vi "sub_calibrate sensor data.vi"(1 "Sensor Column":i32, 2 "Raw Data":dbl) -> (0 "Calibrated Data":dbl)   [LabVIEW 2021]
uses:
  globalvariables.vi
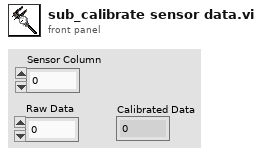
[diagram p1: front panel]
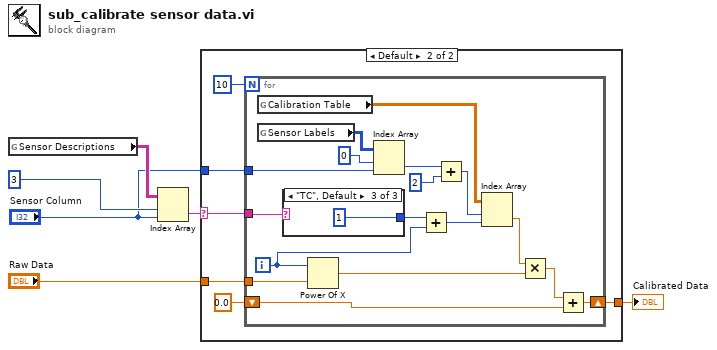
[diagram p0: block diagram]
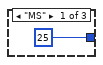
[diagram p3: hidden frame]
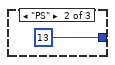
[diagram p4: hidden frame]
diagram:
  n1 = global read "globalvariables.vi" "Sensor Descriptions"() -> (w3:string[][])
  n2 = Index Array(array=w3, index (row)=3, index (col)="Sensor Column") -> (element=w1:string)
  n3 = case shown="Default" w1 {
    selector: w1 -> [_ w9]
    tunnel: [w7 w12] -> w6
    tunnel: "Raw Data" -> [w7 w10]
    tunnel: "Sensor Column" -> [_ w11]
    frame "TM" {
    }
    frame Default {
      n4 = for {
        N: 10 -> [_]
        shift-right: [w30] -> w12
        shift-left: 0.0 -> [w29]
        tunnel: w10 -> [w28]
        tunnel: w11 -> [w27]
        tunnel: w9 -> [w16]
        i -> [w14]
        n5 = global read "globalvariables.vi" "Calibration Table"() -> (w22:dbl[][])
        n6 = global read "globalvariables.vi" "Sensor Labels"() -> (w23:i32[][])
        n7 = case shown="\"TC\", Default" w16 {
          tunnel: [25 13 1] -> w15
          frame "MS" {
          }
          frame "PS" {
          }
          frame "TC", Default {
          }
        }
        n8 = Power Of X(1:w28, 2:w14) -> (0:w26:dbl)
        n9 = Index Array(array=w23, index (row)=0, index (col)=w27) -> (element=w18:i32)
        n10 = Add(x=w15, y=w14) -> (x+y=w20:i32)
        n11 = Add(x=w18, y=2) -> (x+y=w19:i32)
        n12 = Index Array(array=w22, index (row)=w19, index (col)=w20) -> (element=w24:dbl)
        n13 = Multiply(x=w24, y=w26) -> (x*y=w25:dbl)
        n14 = Add(x=w25, y=w29) -> (x+y=w30:dbl)
      }
    }
  }
  "Calibrated Data" <- w6
